vi "Grab.vi"(8 "error in (no error)":errorcluster, 10 "Image in":T1, 11 "IMAQ Camera in":refnum<class "IMAQ Camera.lvclass">) -> (0 "error out":errorcluster, 2 "Image out":T1, 3 "IMAQ Camera out":refnum<class "IMAQ Camera.lvclass">)   [LabVIEW 2011, in "IMAQ Camera.lvclass"]
uses:
  IMAQ Camera.lvclass
  <vilib>/vision/Image Controls.llb/IMAQ Image.ctl
  IMAQ Camera.lvclass/IMAQ Camera.ctl
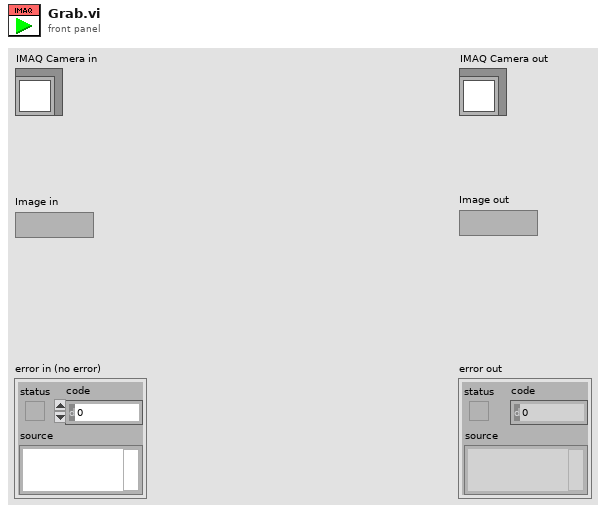
[diagram p1: front panel]
types:
  T1 = typedef "IMAQ Image.ctl" = refnum<image>
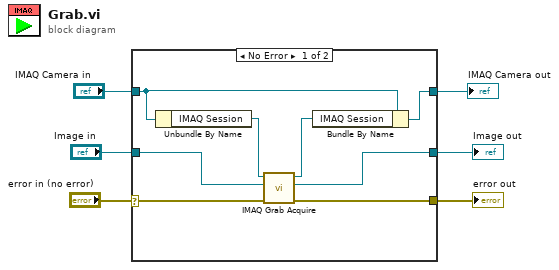
[diagram p0: block diagram]
diagram:
  n1 = case shown="No Error" "error in (no error)" {
    selector: "error in (no error)" -> [w7 w16]
    tunnel: "Image in" -> [w13 w17]
    tunnel: [w12 w16] -> w5
    tunnel: [w11 w17] -> w4
    tunnel: "IMAQ Camera in" -> [w9 w15]
    tunnel: [w8 w15] -> w2
    frame No Error {
      n2 = Unbundle By Name(w9) -> ("IMAQ Session"=w14:refnum<k11>)
      n3 = call <vilib>:"IMAQ Grab Acquire.vi"("error in (no error)"=w7, "Image In"=w13, "IMAQ Session In"=w14) -> ("error out"=w12:errorcluster, "Image Out"=w11:T1, "IMAQ Session Out"=w10:refnum<k11>)  [unwired: 5 in, 1 out]
      n4 = Bundle By Name(cluster=w9, "IMAQ Session"=w10) -> (w8:refnum<class "IMAQ Camera.lvclass">)
    }
    frame Error {
    }
  }
  "error out" <- w5
  "IMAQ Camera out" <- w2
  "Image out" <- w4
